vi "FGV Data.vi"(7 "Action":enum16{"Initial", "Read", "Write"}(ring), 8 "error in (no error)":errorcluster caption="错误输入（无错误）", 11 "Data IN":cluster{"Con?":bool, "温度":dbl[]}) -> (0 "error out":errorcluster caption="错误输出", 3 "Data OUT":cluster{"Con?":bool, "温度":dbl[]})   [LabVIEW 2018]
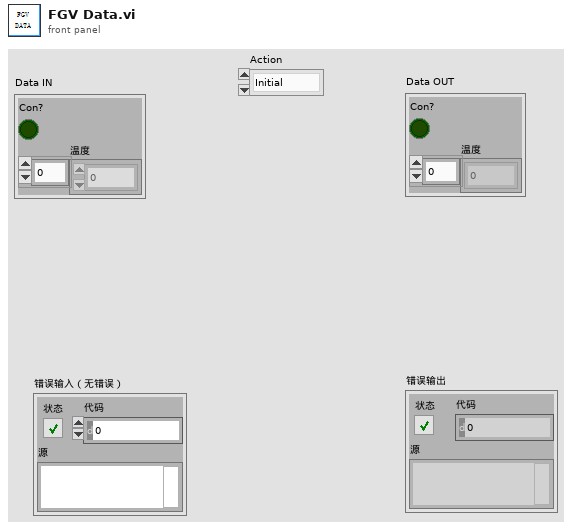
[diagram p1: front panel]
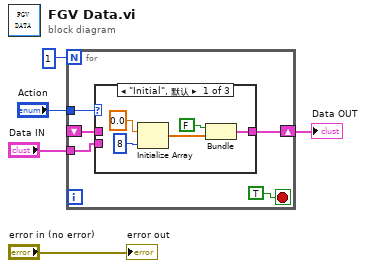
[diagram p0: block diagram]
diagram:
  n1 = for {
    N: 1 -> [_]
    tunnel: "Action" -> [w9]
    shift-right: [w8] -> w2
    shift-left: _ -> [w7]
    tunnel: "Data IN" -> [w6]
    stop <- TRUE stop-if-true
    n2 = case shown="\"Initial\", 默认" w9 {
      tunnel: [w13 w16 w17] -> w8
      tunnel: w7 -> [_ w16 _]
      tunnel: w6 -> [_ _ w17]
      frame "Initial", Default {
        n3 = Initialize Array(0.0, 8 ("维数大小")) -> (w12:dbl[])
        n4 = Bundle(FALSE, w12) -> (w13:cluster{bool, dbl[]})  [unwired: 1 in]
      }
      frame "Read" {
      }
      frame "Write" {
      }
    }
  }
  "Data OUT" <- w2
  "error out" <- "error in (no error)"
